vi "Create Polynomial From Conjugate Roots.vi"(11 "Conjugate Complex":cdb[](array[numeric])) -> (3 "P(x)":dbl[](array[numeric]))   [LabVIEW 2020, in "NI_AALPro.lvlib"]
uses:
  <vilib>/Analysis/NI_AALPro.lvlib
  <vilib>/Analysis/polynomials.llb/Leja Order Roots (CDB).vi
  <vilib>/Analysis/polynomials.llb/Multiply Polynomials (DBL).vi
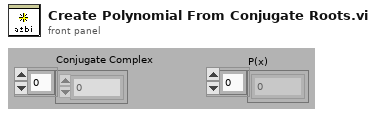
[diagram p1: front panel]
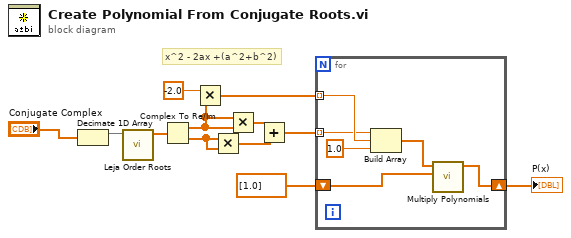
[diagram p0: block diagram]
diagram:
  # "x^2 - 2ax +(a^2+b^2)"
  n1 = Decimate 1D Array("Conjugate Complex") -> (w2:cdb[])  [unwired: 1 out]
  n2 = call-poly <vilib>:"Leja Order Roots.vi"("Roots"=w2) -> ("Roots of Leja Order"=w1:cdb[])  [unwired: 10 in]
  n3 = Complex To Re/Im(x + iy=w1) -> (x=w10:dbl[], y=w9:dbl[])
  n4 = Multiply(x=-2.0, y=w10) -> (x*y=w5:dbl[])
  n5 = Multiply(x=w9, y=w9) -> (x*y=w7:dbl[])
  n6 = Multiply(x=w10, y=w10) -> (x*y=w8:dbl[])
  n7 = Add(x=w8, y=w7) -> (x+y=w6:dbl[])
  n8 = for {
    shift-right: [w13] -> w3
    shift-left: dbl[] [1.0] -> [w14]
    tunnel: w6 -> [w17] mode=indexing
    tunnel: w5 -> [w18] mode=indexing
    n9 = Build Array(w17, w18, 1.0 ("element")) -> (w15:dbl[])
    n10 = call-poly <vilib>:"Multiply Polynomials.vi"("Q(x)"=w14, "P(x)"=w15) -> ("P(x)*Q(x)"=w13:dbl[])  [unwired: 8 in, 1 out]
  }
  "P(x)" <- w3
